vi "Sysdef.SimpleExport.vi"(8 "error in (no error)":errorcluster, 11 "ID":u64) -> (0 "error out":errorcluster, 2 "Export":T1 {"Tree"."Properties"."Type" items=["K_STRING", "K_BOOL", "K_I32", "K_U32", "K_DOUBLE", "K_U64", "K_VARIANT", "K_DEPENDENTFILE", "K_DEPENDENTNODE", "K_DATASOURCENODE", "K_U16", "K_DBLARR", "K_U32ARR", "K_I32ARR", "K_STRINGARR", "K_DICTIONARY", "K_DICTIONARYARR"]}, 3 "ID out":u64)   [LabVIEW 2020, in "ImportExport.lvlib"]
doc: "Uses the NI VeriStand .NET API to save the Custom Device Hierarchy (Sections, Channels, Waveforms) as well as its Items Properties into a cluster."
uses:
  ImportExport.lvlib
  <vilib>/NI/NI VeriStand Advanced SysDef API/_Types/SysDef.Export.ctl
  <vilib>/NI/NI VeriStand Advanced SysDef API/_Types/TreeItem.ctl
  <vilib>/NI/NI VeriStand Advanced SysDef API/_Types/TreeItem.Info.ctl
  <vilib>/NI VeriStand/Custom Device API/Custom Device Channel.ctl
  <vilib>/NI VeriStand/Custom Device API/Custom Device Channel Type.ctl
  <vilib>/NI VeriStand/Custom Device API/Custom Device Waveform.ctl
  <vilib>/NI VeriStand/Custom Device API/Custom Device Waveform DataType.ctl
  <vilib>/NI/NI VeriStand Advanced SysDef API/_Types/TreeItem.Property.ctl
  NationalInstruments.VeriStand.SystemDefinitionAPI
  <vilib>/NI/NI VeriStand Advanced SysDef API/SysDef API/Advanced System Definition.lvlib
  <vilib>/NI VeriStand/Custom Device API/Custom Device API.lvlib
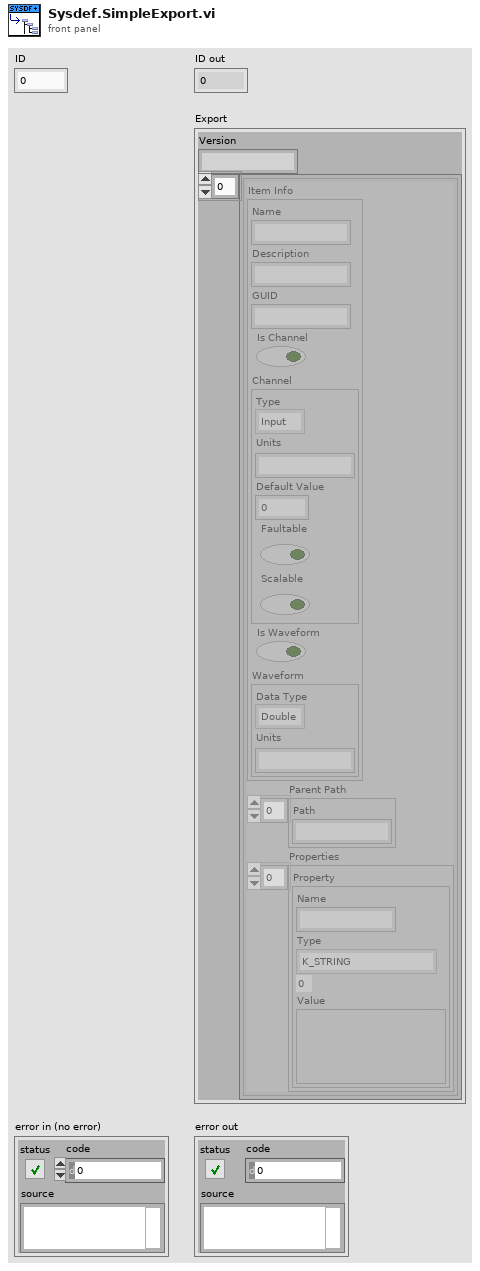
[diagram p1: front panel]
types:
  T1 = typedef "Advanced System Definition.lvlib/SysDef.Export.ctl" = cluster{"Version":string, "Tree":T2[]}
  T2 = typedef "Advanced System Definition.lvlib/TreeItem.ctl" = cluster{"Item Info":T3, "Parent Path":string[], "Properties":T8[]}
  T3 = typedef "Advanced System Definition.lvlib/TreeItem.Info.ctl" = cluster{"Name":string, "Description":string, "GUID":string, "Is Channel":bool, "Channel":T4, "Is Waveform":bool, "Waveform":T6}
  T4 = typedef "Custom Device API.lvlib/Custom Device Channel.ctl" = cluster{"Type":T5, "Units":string, "Default Value":dbl, "Faultable":bool, "Scalable":bool}
  T5 = typedef "Custom Device API.lvlib/Custom Device Channel Type.ctl" = enum16{"Input", "Output"}
  T6 = typedef "Custom Device API.lvlib/Custom Device Waveform.ctl" = cluster{"Data Type":T7, "Units":string}
  T7 = typedef "Custom Device API.lvlib/Custom Device Waveform DataType.ctl" = enum16{"Double", "Complex Double"}
  T8 = typedef "Advanced System Definition.lvlib/TreeItem.Property.ctl" = cluster{"Name":string, "Type":i32, "Value":variant}
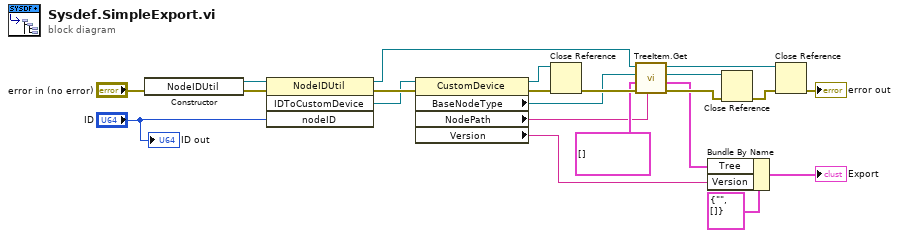
[diagram p0: block diagram]
diagram:
  n1 = constructor class="NodeIDUtil"(error in="error in (no error)") -> (reference out=w17:refnum<k24>, error out=w19:errorcluster)  [unwired: 2 in, 1 out]
  n2 = invoke class="NodeIDUtil" method="IDToCustomDevice"(reference=w17, error in=w19, "nodeID"="ID") -> (reference out=w12:refnum<k24>, error out=w22:errorcluster, "IDToCustomDevice"=w21:refnum<k24>)  [unwired: 1 in, 1 out]
  n3 = property class="CustomDevice"(reference=w21, error in=w22) -> (reference out=w14:refnum<k24>, error out=w16:errorcluster, "BaseNodeType"=w13:refnum<k24>, "NodePath"=w1:string, "Version"=w4:string)
  n4 = Close Reference(reference=w14, error in (no error)=w16) -> (error out=w15:errorcluster)
  n5 = call <vilib>:"TreeItem.Get.vi"("Custom Device Path"=w1, "error in (no error)"=w15, "Tree"=T2[] [], "BaseNode Ref"=w13, "NodeIDUtil Ref"=w12) -> ("error out"=w10:errorcluster, "Tree"=w2:T2[], "BaseNode Ref out"=w11:refnum<k24>, "NodeIDUtil Ref out"=w7:refnum<k24>)  [unwired: 3 in]
  n6 = Bundle By Name(cluster=T1 {"Version"="", "Tree"=[]}, "Tree"=w2, "Version"=w4) -> (→"Export":T1)
  n7 = Close Reference(reference=w11, error in (no error)=w10) -> (error out=w9:errorcluster)
  n8 = Close Reference(reference=w7, error in (no error)=w9) -> (error out=→"error out":errorcluster)
  "ID out" <- "ID"
